vi "Destroy.vi"(8 "error in (no error)":errorcluster, 11 "Tetris in":refnum<class "Tetris.lvclass">) -> (0 "error out":errorcluster, 3 "FPGA_ref":T1)   [LabVIEW 2019, in "RT_Game.lvlib" / "Tetris.lvclass"]
uses:
  Tetris.lvclass
  FPGA_Interface.ctl
  Game/Game.lvclass
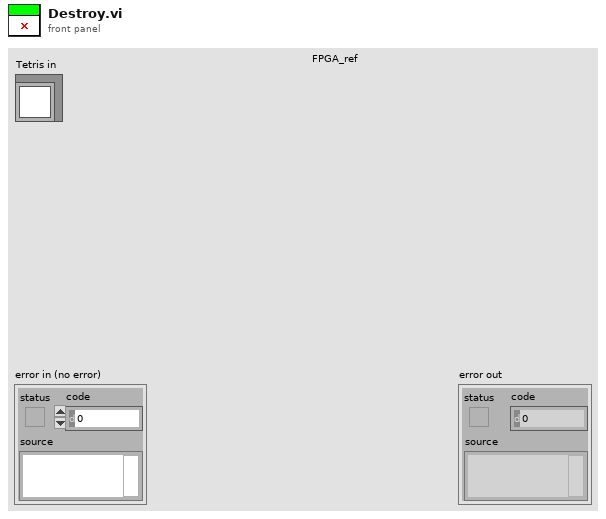
[diagram p1: front panel]
types:
  T1 = typedef "FPGA_Interface.ctl" = refnum<k20>
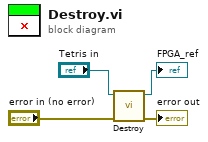
[diagram p0: block diagram]
diagram:
  n1 = call-parent "Destroy.vi"("error in (no error)"="error in (no error)", "Game in"="Tetris in") -> ("error out"=→"error out":errorcluster, "FPGA_ref"=→"FPGA_ref":T1)  [unwired: 8 in]
